vi "Merge Status.vi"(10 "New":T1, 11 "Current":T1) -> (1 "Changed?":bool, 3 "Merged":T1)   [LabVIEW 2020, in "Test Suite Result.lvlib"]
uses:
  Test Suite Result.lvlib
  Assertion Result/Public/TypeDefs/Status.ctl
  Assertion Result/Assertion Result.lvlib
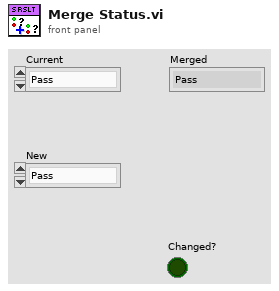
[diagram p1: front panel]
types:
  T1 = typedef "Assertion Result.lvlib/Status.ctl" = enum16{"Pass", "Fail", "Error", "Skipped", "Setup Error", "Broken", "Teardown Error"}
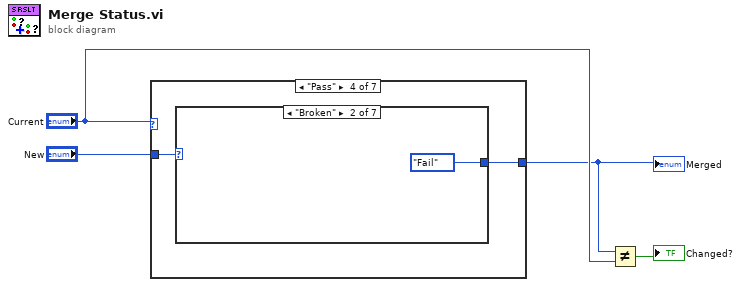
[diagram p0: block diagram]
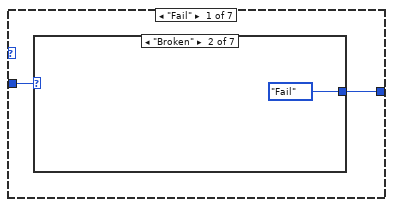
[diagram p2: hidden frame]
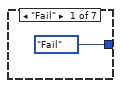
[diagram p3: hidden frame]
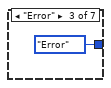
[diagram p4: hidden frame]
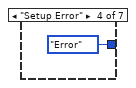
[diagram p5: hidden frame]
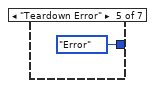
[diagram p6: hidden frame]
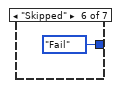
[diagram p7: hidden frame]
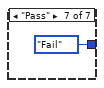
[diagram p8: hidden frame]
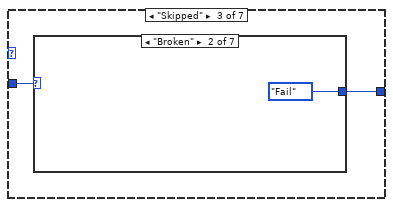
[diagram p10: hidden frame]
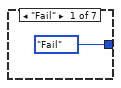
[diagram p11: hidden frame]
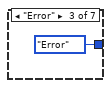
[diagram p12: hidden frame]
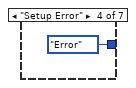
[diagram p13: hidden frame]
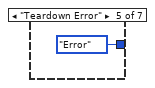
[diagram p14: hidden frame]
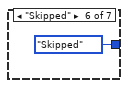
[diagram p15: hidden frame]
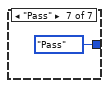
[diagram p16: hidden frame]
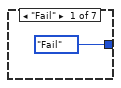
[diagram p17: hidden frame]
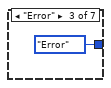
[diagram p18: hidden frame]
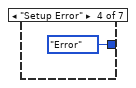
[diagram p19: hidden frame]
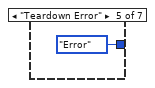
[diagram p20: hidden frame]
diagram:
  n1 = case shown="\"Pass\"" "Current" {
    tunnel: "New" -> [w6 w14 w16 w25 _ _ _]
    tunnel: [w5 w14 w15 w24 Status."Error" ("Merged Status") Status."Error" ("Merged Status") Status."Error" ("Merged Status")] -> w2
    frame "Fail" {
      n2 = case shown="\"Broken\"" w6 {
        tunnel: [Status."Fail" ("Merged Status") Status."Fail" ("Merged Status") Status."Error" ("Merged Status") Status."Error" ("Merged Status") Status."Error" ("Merged Status") Status."Fail" ("Merged Status") Status."Fail" ("Merged Status")] -> w5
        frame "Fail" {
        }
        frame "Broken" {
        }
        frame "Error" {
        }
        frame "Setup Error" {
        }
        frame "Teardown Error" {
        }
        frame "Skipped" {
        }
        frame "Pass" {
        }
      }
    }
    frame "Broken" {
    }
    frame "Skipped" {
      n3 = case shown="\"Broken\"" w16 {
        tunnel: [Status."Fail" ("Merged Status") Status."Fail" ("Merged Status") Status."Error" ("Merged Status") Status."Error" ("Merged Status") Status."Error" ("Merged Status") Status."Skipped" ("Merged Status") Status."Pass" ("Merged Status")] -> w15
        frame "Fail" {
        }
        frame "Broken" {
        }
        frame "Error" {
        }
        frame "Setup Error" {
        }
        frame "Teardown Error" {
        }
        frame "Skipped" {
        }
        frame "Pass" {
        }
      }
    }
    frame "Pass" {
      n4 = case shown="\"Broken\"" w25 {
        tunnel: [Status."Fail" ("Merged Status") Status."Fail" ("Merged Status") Status."Error" ("Merged Status") Status."Error" ("Merged Status") Status."Error" ("Merged Status") Status."Pass" ("Merged Status") Status."Pass" ("Merged Status")] -> w24
        frame "Fail" {
        }
        frame "Broken" {
        }
        frame "Error" {
        }
        frame "Setup Error" {
        }
        frame "Teardown Error" {
        }
        frame "Skipped" {
        }
        frame "Pass" {
        }
      }
    }
    frame "Error" {
    }
    frame "Setup Error" {
    }
    frame "Teardown Error" {
    }
  }
  "Merged" <- w2
  n5 = Not Equal?(x=w2, y="Current") -> (x != y?=→"Changed?":bool)
